vi "Configure Electrical Delay.vi"(0 "VISA resource name":refnum<visa-resource-name>, 1 "Unit (0: Meter)":i32(ring) items=["Meter", "Feet", "Inch"], 2 "Waveguide Cutoff Frequency (4.5E+7 Hz)":dbl=45000000.0, 5 "Channel (1)":i32=1, 7 "Distance (0)":dbl, 9 "Medium (0: Coaxial)":i32(ring) items=["Coaxial", "Waveguide"], 11 "error in (no error)":errorcluster, 12 "Delay (0 s)":dbl) -> (4 "VISA resource name out":refnum<visa-resource-name>, 15 "error out":errorcluster)   [LabVIEW 2018, in "Keysight PNA Series.lvlib"]
doc: "Configures the electrical delay."
uses:
  Keysight PNA Series.lvlib
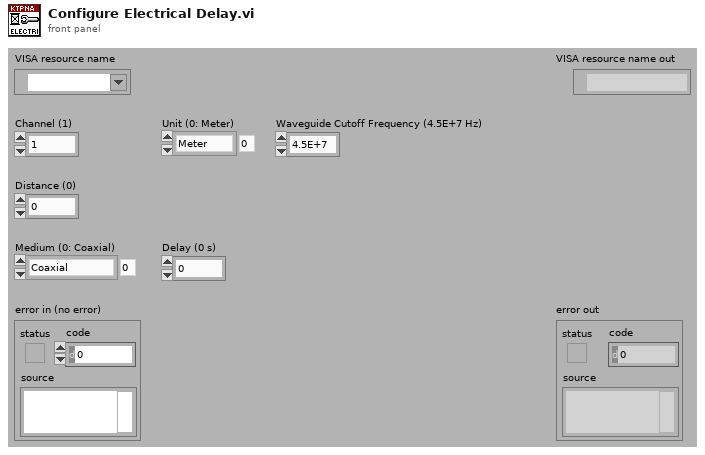
[diagram p1: front panel]
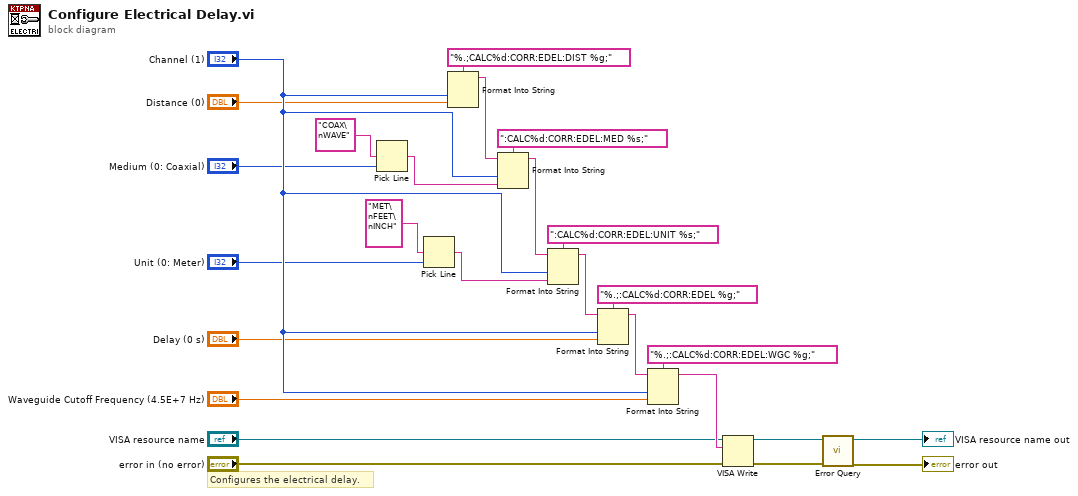
[diagram p0: block diagram]
diagram:
  # "Configures the electrical delay."
  n1 = Pick Line(multi-line string="COAX\nWAVE", line index="Medium (0: Coaxial)") -> (output string=w19:string)  [unwired: 1 in]
  n2 = Pick Line(multi-line string="MET\nFEET\nINCH", line index="Unit (0: Meter)") -> (output string=w14:string)  [unwired: 1 in]
  n3 = Format Into String(format string="%.;CALC%d:CORR:EDEL:DIST %g;", "Channel (1)", "Distance (0)") -> (resulting string=w21:string)  [unwired: 2 in, 1 out]
  n4 = Format Into String(format string=":CALC%d:CORR:EDEL:MED %s;", initial string=w21, "Channel (1)", w19) -> (resulting string=w16:string)  [unwired: 1 in, 1 out]
  n5 = Format Into String(format string=":CALC%d:CORR:EDEL:UNIT %s;", initial string=w16, "Channel (1)", w14) -> (resulting string=w13:string)  [unwired: 1 in, 1 out]
  n6 = Format Into String(format string="%.;:CALC%d:CORR:EDEL %g;", initial string=w13, "Channel (1)", "Delay (0 s)") -> (resulting string=w10:string)  [unwired: 1 in, 1 out]
  n7 = Format Into String(format string="%.;:CALC%d:CORR:EDEL:WGC %g;", initial string=w10, "Channel (1)", "Waveguide Cutoff Frequency (4.5E+7 Hz)") -> (resulting string=w7:string)  [unwired: 1 in, 1 out]
  n8 = VISA Write(VISA resource name="VISA resource name", write buffer=w7, error in (no error)="error in (no error)") -> (VISA resource name out=w4:refnum<visa-resource-name>, error out=w3:errorcluster)  [unwired: 1 out]
  n9 = call "Error Query.vi"("error in (no error)"=w3, "VISA resource name"=w4) -> ("error out"=→"error out":errorcluster, "VISA resource name out"=→"VISA resource name out":refnum<visa-resource-name>)  [unwired: 6 in, 2 out]
